vi "2D Array an Zeile x bis zum leren Element.vi"(10 "Index (Zeile)":i32, 11 "Part Array":string[][](array[string])) -> (3 "Array gestutzt":string[][](array[string]))   [LabVIEW 2020, in "Linearisierung v2.lvlib" / "SpanEinstellungen.lvlib"]
uses:
  SpanEinstellungen.lvlib
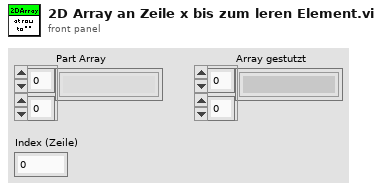
[diagram p1: front panel]
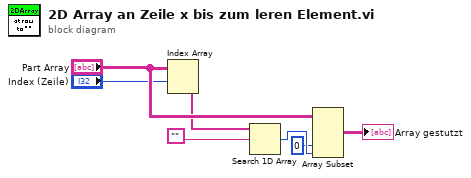
[diagram p0: block diagram]
diagram:
  n1 = Index Array(array="Part Array", index (row)="Index (Zeile)") -> (element=w2:string[])  [unwired: 1 in]
  n2 = Search 1D Array(1D array=w2, element="") -> (index of element=w5:i32)  [unwired: 1 in]
  n3 = Array Subset(array="Part Array", index (col)=0 ("Index"), length (col)=w5) -> (→"Array gestutzt":string[][])  [unwired: 2 in]
